vi "Parse Serial Data String.vi"(5 "delimiter":string, 6 "serial data string":string) -> (2 "parsed serial data":T1)   [LabVIEW 2025]
uses:
  Serial Data.ctl
  <vilib>/Utility/error.llb/Trim Whitespace One-Sided.vi
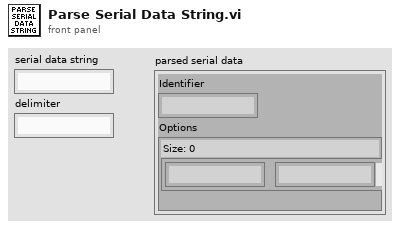
[diagram p1: front panel]
types:
  T1 = typedef "Serial Data.ctl" = cluster{"Identifier":string, "Options":map{string, string}}
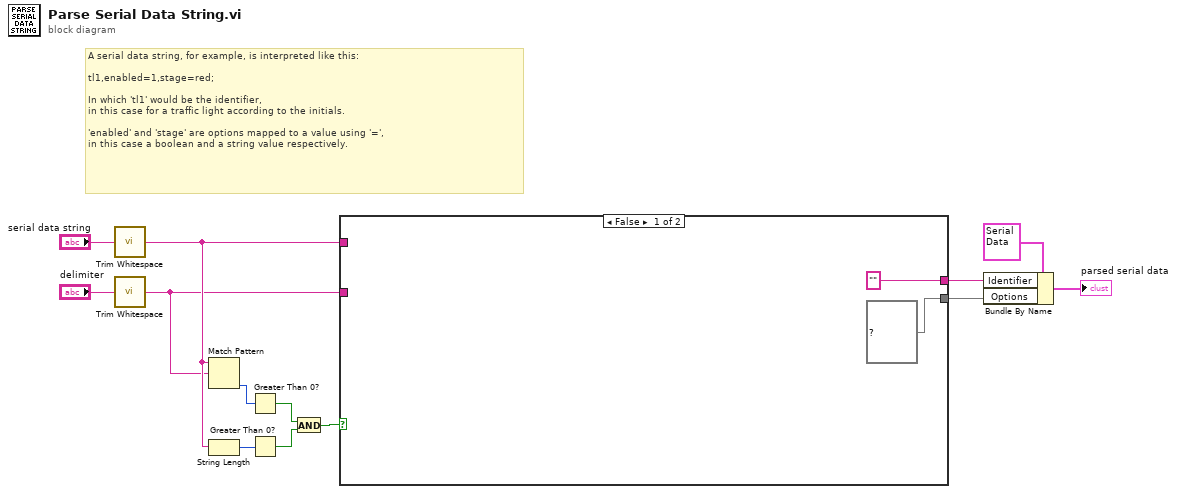
[diagram p0: block diagram]
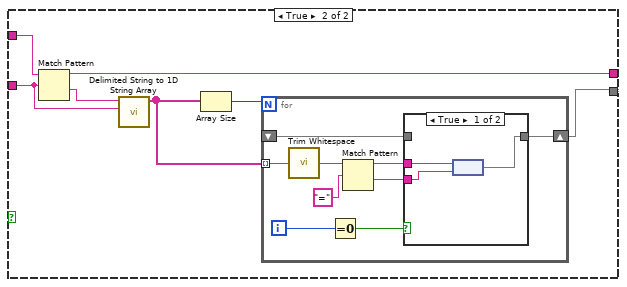
[diagram p2: hidden frame]
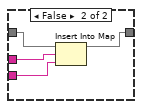
[diagram p3: hidden frame]
diagram:
  # "A serial data string, for example, is interpreted like this:\n\ntl1,enabled=1,stage=red;\n\nIn which 'tl1' would be the identifier,\nin this case for a traffic light according to the initials.\n\n'enabled' and 'stage' are options mapped to a value using '=',\nin this case a boolean and a string value respectively."
  n1 = call <vilib>:"Trim Whitespace.vi"("string"="serial data string") -> ("trimmed string"=w6:string)  [unwired: 1 in]
  n2 = call <vilib>:"Trim Whitespace.vi"("string"="delimiter") -> ("trimmed string"=w5:string)  [unwired: 1 in]
  n3 = Match Pattern(string=w6, regular expression=w5) -> (offset past match=w1:i32)  [unwired: 1 in, 3 out]
  n4 = String Length(string=w6) -> (length=w11:i32)
  n5 = Greater Than 0?(x=w1) -> (x > 0?=w2:bool)
  n6 = Greater Than 0?(x=w11) -> (x > 0?=w3:bool)
  n7 = And(x=w2, y=w3) -> (x .and. y?=w4:bool)
  n8 = case shown="False" w4 {
    tunnel: w6 -> [_ w19]
    tunnel: w5 -> [_ w18]
    tunnel: ["" ("trimmed string") w17] -> w8
    tunnel: [map{string, string} {} ("map") w16] -> w7
    frame False {
    }
    frame True {
      n9 = Match Pattern(string=w19, regular expression=w18) -> (before substring=w17:string, after substring=w22:string)  [unwired: 1 in, 2 out]
      n10 = call <vilib>:"Delimited String to 1D String Array.vi"("delimiter"=w18, "delimited string"=w22) -> ("string array"=w20:string[])  [unwired: 9 in]
      n11 = Array Size(array=w20) -> (size(s)=w21:i32)
      n12 = for {
        N: w21 -> [_]
        tunnel: w20 -> [w30] mode=indexing
        shift-right: [w24] -> w16
        shift-left: _ -> [w23]
        i -> [w26]
        n13 = call <vilib>:"Trim Whitespace.vi"("string"=w30) -> ("trimmed string"=w29:string)  [unwired: 1 in]
        n14 = Equal To 0?(x=w26) -> (x = 0?=w27:bool)
        n15 = Match Pattern(string=w29, regular expression="=") -> (before substring=w28:string, after substring=w25:string)  [unwired: 1 in, 2 out]
        n16 = case shown="True" w27 {
          tunnel: w28 -> [w34 w36]
          tunnel: [w33 w37] -> w24
          tunnel: w25 -> [w32 w35]
          tunnel: w23 -> [_ w38]
          frame True {
            n17 = node(w34, w32) -> (w33:map{string, string})
          }
          frame False {
            n18 = Insert Into Map(map in=w38, key=w36, value=w35) -> (map out=w37:map{string, string})  [unwired: 2 out]
          }
        }
      }
    }
  }
  n19 = Bundle By Name(cluster=T1 {"Identifier"="", "Options"={}} ("Serial Data"), "Identifier"=w8, "Options"=w7) -> (→"parsed serial data":T1)
